vi "String_Find many Strings.vi"(10 "Target":string, 11 "Target List":string[](array[string])) -> (2 "Exact Match Out":bool[](array[boolean]), 3 "Index Out":i32[](array[numeric]))   [LabVIEW 2023]
uses:
  daaa9eff-712e-497d-ae34-0a6b443bd322.vi
  b6a16de6-4b00-4e98-8248-8915008b39a1.vi
  daaa9eff-712e-497d-ae34-0a6b443bd322.vi/86a48f32-e87b-45aa-832a-4b8f4efc5d94.vi
  b6a16de6-4b00-4e98-8248-8915008b39a1.vi/81b768ac-65a2-4ca0-9267-587cf97d9e49.vi
  <vilib>/Utility/error.llb/Trim Whitespace.vi
  <vilib>/Utility/error.llb/Trim Whitespace One-Sided.vi
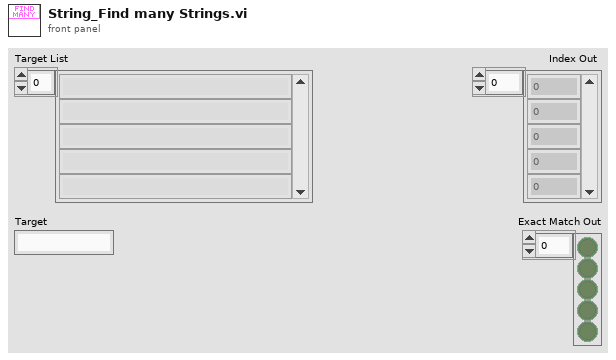
[diagram p1: front panel]
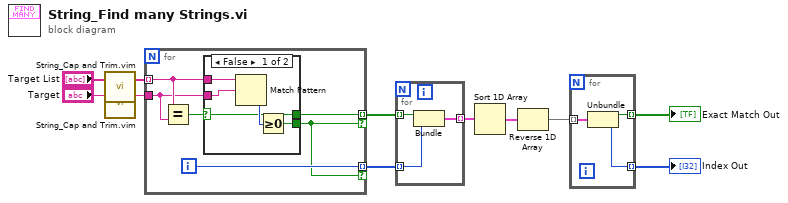
[diagram p0: block diagram]
diagram:
  n1 = call "String_Cap and Trim.vim"("String In"="Target List") -> ("String Array Out"=w9:string[])  [unwired: 2 in]
  n2 = call "String_Cap and Trim.vim"("String In"="Target") -> ("String Array Out"=w10:string)  [unwired: 2 in]
  n3 = for {
    tunnel: w9 -> [w17] mode=indexing
    tunnel: w10 -> [w16]
    tunnel: [w14] -> w8 mode=indexing if=w12
    tunnel: [w13] -> w7 mode=indexing if=w12
    i -> [w13]
    n4 = Equal?(x=w17, y=w16) -> (x = y?=w15:bool)
    n5 = case shown="False" w15 {
      selector: w15 -> [w18 w23]
      tunnel: w17 -> [w22 _]
      tunnel: w16 -> [w21 _]
      tunnel: [w18 w23] -> w14
      tunnel: [w19 w23] -> w12
      frame False {
        n6 = Match Pattern(string=w22, regular expression=w21) -> (offset past match=w20:i32)  [unwired: 1 in, 3 out]
        n7 = Greater Or Equal To 0?(x=w20) -> (x >= 0?=w19:bool)
      }
      frame True {
      }
    }
  }
  n8 = for {
    tunnel: w7 -> [w25] mode=indexing
    tunnel: w8 -> [w26] mode=indexing
    tunnel: [w24] -> w3 mode=indexing
    n9 = Bundle(w26, w25) -> (w24:cluster{bool, i32})  [unwired: 1 in]
  }
  n10 = Sort 1D Array(array=w3) -> (sorted array=w2:cluster{bool, i32}[])
  n11 = Reverse 1D Array(array=w2) -> (reversed array=w1:cluster{bool, i32}[])
  n12 = for {
    tunnel: w1 -> [w29] mode=indexing
    tunnel: [w28] -> w6 mode=indexing
    tunnel: [w27] -> w5 mode=indexing
    n13 = Unbundle(w29) -> (w28:bool, w27:i32)
  }
  "Index Out" <- w5
  "Exact Match Out" <- w6
